vi "sub_Initialize.vi"(8 "error in":errorcluster caption="에러 입력", 10 "Car Position Slider":refnum<vi>, 11 "Wash Options":refnum<vi>) -> (0 "error out":errorcluster caption="에러 출력")   [LabVIEW 2017]
uses:
  Control/Wash Options.ctl
  Control/Car Position Control.ctl
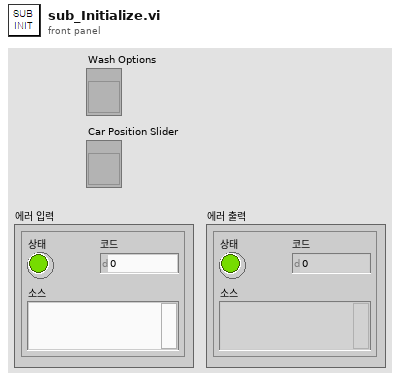
[diagram p1: front panel]
types:
  T1 = enum8{"Enabled", "Disabled", "Disabled and Grayed Out"}
  T2 = typedef "Car Position Control.ctl" = i32
  T3 = typedef "Wash Options.ctl" = cluster{"Under Body Wash":bool, "Bug Remover":bool, "Pre-Soak":bool, "High Pressure Wash":bool, "Low Pressure Wax":bool, "Spot Free Rinse":bool, "Tire Shine Foam":bool, "Air Dry":bool}
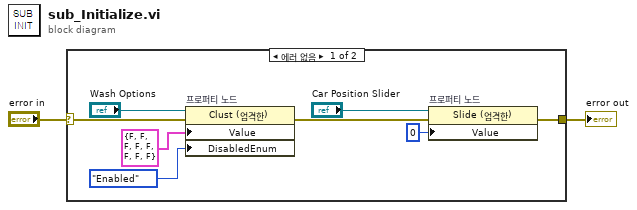
[diagram p0: block diagram]
diagram:
  n1 = case shown="에러 없음" "error in" {
    selector: "error in" -> [w3 w11]
    tunnel: [w6 w11] -> w1
    frame No Error {
      n2 = property on="프로퍼티 노드" class="Clust (엄격한)"(reference="Wash Options", error in=w3, "Value"=T3 {"Under Body Wash"=FALSE, "Bug Remover"=FALSE, "Pre-Soak"=FALSE, "High Pressure Wash"=FALSE, "Low Pressure Wax"=FALSE, "Spot Free Rinse"=FALSE, "Tire Shine Foam"=FALSE, "Air Dry"=FALSE} ("값"), "DisabledEnum"=T1."Enabled" ("비활성화")) -> (error out=w8:errorcluster)  [unwired: 1 out]
      n3 = property on="프로퍼티 노드" class="Slide (엄격한)"(reference="Car Position Slider", error in=w8, "Value"=T2 0 ("값")) -> (error out=w6:errorcluster)  [unwired: 1 out]
    }
    frame Error {
    }
  }
  "error out" <- w1
